vi "WriteCANFrame.vi"(6 "Log Data?":bool, 8 "error in (no error)":errorcluster, 9 "timeout (10)":dbl=10.0 format="%.2g", 10 "data":T1[](array[typedef]) {"payload" format="%x"; "timestamp" format="%<%.7X\n%x>T"; "type" items=["CAN Data"=0, "CAN Remote"=1, "CAN Bus Error"=2, "CAN 2.0 Data"=8, "CAN FD Data"=16, "CAN FD+BRS Data"=24, "J1939 Data"=192, "Delay"=224, "Log Trigger"=225, "Start Trigger"=226]; "identifier" format="%x"}, 11 "NI-XNET in":refnum<class "NI-XNET.lvclass">) -> (0 "error out":errorcluster, 3 "NI-XNET out":refnum<class "NI-XNET.lvclass">)   [LabVIEW 2023, in "HardwareAbstractionLayer_LVOOP.lvlib" / "CAN HAL Lib.lvlib" / "NI-XNET.lvclass"]
uses:
  NI-XNET.lvclass
  <vilib>/xnet/xnet.llb/XNET Frame CAN.ctl
  <vilib>/xnet/xnet.llb/XNET Frame Type CAN.ctl
  NI-XNET.lvclass/NI-XNET.ctl
  <vilib>/xnet/xnet.llb/XNET Write (Frame CAN).vi
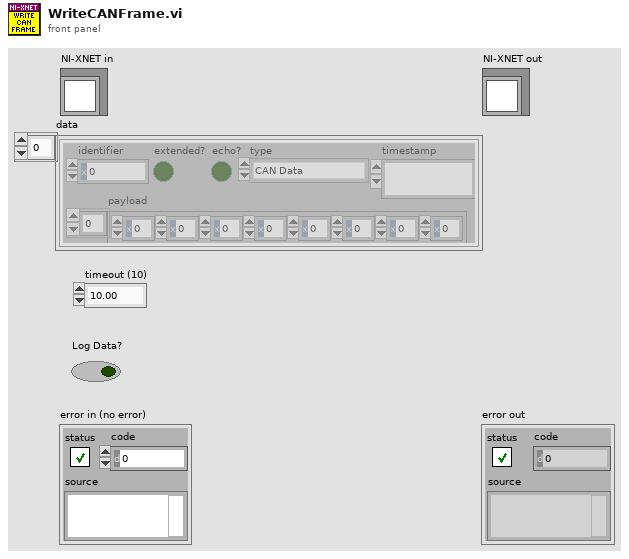
[diagram p1: front panel]
types:
  T1 = typedef "XNET Frame CAN.ctl" = cluster{"timestamp":timestamp, "payload":u8[], "identifier":u32, "type":T2, "extended?":bool, "echo?":bool}
  T2 = typedef "XNET Frame Type CAN.ctl" = u8
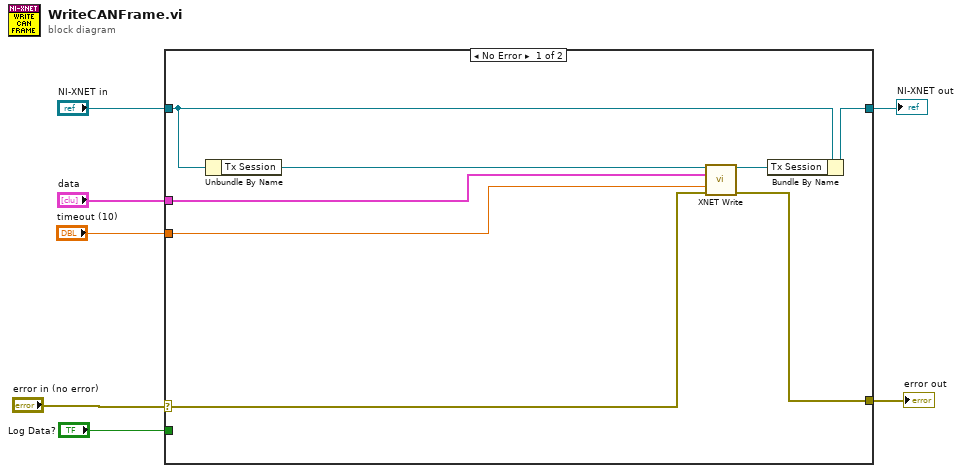
[diagram p0: block diagram]
diagram:
  n1 = case shown="No Error" "error in (no error)" {
    selector: "error in (no error)" -> [w10 w17]
    tunnel: [w13 w17] -> w5
    tunnel: [w12 w16] -> w7
    tunnel: "NI-XNET in" -> [w15 w16]
    tunnel: "data" -> [w9 _]
    tunnel: "timeout (10)" -> [w8 _]
    tunnel: "Log Data?" -> [_ _]
    frame No Error {
      n2 = Unbundle By Name(w15) -> ("Tx Session"=w14:refnum<k21>)
      n3 = call-poly <vilib>:"XNET Write.vi"("session in"=w14, "data"=w9, "timeout (10)"=w8, "error in (no error)"=w10) -> ("session out"=w11:refnum<k21>, "error out"=w13:errorcluster)  [unwired: 10 in]
      n4 = Bundle By Name(cluster=w15, "Tx Session"=w11) -> (w12:refnum<class "NI-XNET.lvclass">)
    }
    frame Error {
    }
  }
  "error out" <- w5
  "NI-XNET out" <- w7
